vi "DEBUG Read Node Classes.vi"(8 "error in (no error)":errorcluster, 11 "Root Node DVR":T1) -> (0 "error out":errorcluster, 3 "Node Classes":string)   [LabVIEW 2015, in "Configuration Tool.lvlib"]
uses:
  Configuration Tool.lvlib
  <vilib>/NI/Configuration Framework/Node/NodeRef.ctl
  <vilib>/NI/Configuration Framework/Node/NISE_CEF_Node.lvclass
  <vilib>/NI/Configuration Framework/Node/NISE_CEF_Node.lvclass/NISE_CEF_Node.ctl
  <vilib>/NI/Configuration Framework/Node/ReadChildren.vi
  <vilib>/NI/Configuration Framework/Node/ReadNodeClass.vi
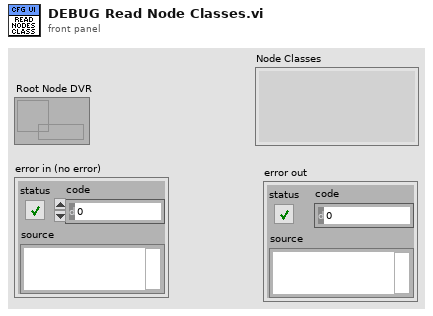
[diagram p1: front panel]
types:
  T1 = typedef "NISE_CEF_Node.lvclass/NodeRef.ctl" = refnum<data-value>
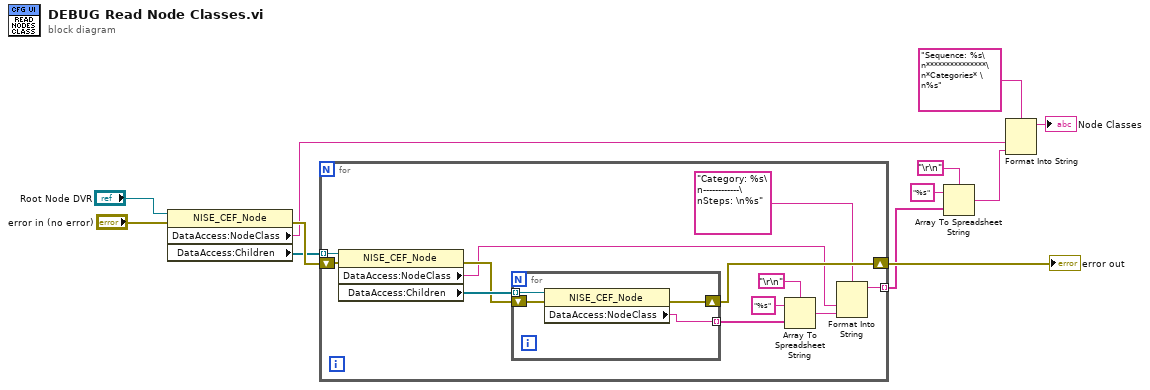
[diagram p0: block diagram]
diagram:
  n1 = property on="Property Node" class="NISE_CEF_Node"(reference="Root Node DVR", error in="error in (no error)") -> (error out=w12:errorcluster, "DataAccess:NodeClass"=w2:string, "DataAccess:Children"=w11:T1[])  [unwired: 1 out]
  n2 = for {
    tunnel: w11 -> [w24] mode=indexing
    shift-right: [w20] -> w8
    shift-left: w12 -> [w23]
    tunnel: [w13] -> w5 mode=indexing
    n3 = property class="NISE_CEF_Node"(reference=w24, error in=w23) -> (error out=w21:errorcluster, "DataAccess:NodeClass"=w15:string, "DataAccess:Children"=w22:T1[])  [unwired: 1 out]
    n4 = for {
      tunnel: w22 -> [w28] mode=indexing
      shift-right: [w26] -> w20
      shift-left: w21 -> [w27]
      tunnel: [w25] -> w17 mode=indexing
      n5 = property class="NISE_CEF_Node"(reference=w28, error in=w27) -> (error out=w26:errorcluster, "DataAccess:NodeClass"=w25:string)  [unwired: 1 out]
    }
    n6 = Array To Spreadsheet String(delimiter (Tab)="\r\n", array=w17, 3:"%s" ("format string")) -> (spreadsheet string=w16:string)
    n7 = Format Into String(format string="Category: %s\n------------\nSteps: \n%s", w15, w16) -> (resulting string=w13:string)  [unwired: 2 in, 1 out]
  }
  "error out" <- w8
  n8 = Array To Spreadsheet String(delimiter (Tab)="\r\n", array=w5, 3:"%s" ("format string")) -> (spreadsheet string=w4:string)
  n9 = Format Into String(format string="Sequence: %s\n***************\n*Categories* \n%s", w2, w4) -> (resulting string=→"Node Classes":string)  [unwired: 2 in, 1 out]
